vi "Query - DBL - 1D - Col.vi"(8 "error in":errorcluster, 10 "Query":string, 11 "Module ID":i32=-1) -> (0 "error out":errorcluster, 1 "Meta Data":variant, 2 "Return Data":dbl[](array[numeric]), 4 "Field Names":string[](array[string]))   [LabVIEW 2022 SP3, in "hse-db.lvlib" / "DB_CONNECTOR.lvlib"]
doc: "returns the first column\n\n____\nHAMPEL SOFTWARE ENGINEERING v1.4.0 (2023-12-19 09:52)"
uses:
  DB_CONNECTOR.lvlib
  hse-libraries/Source/hse-misc/Conversion/ConvertStringToFloat_Array-2D.vi
  hse-libraries/Source/hse-misc/hse-misc.lvlib
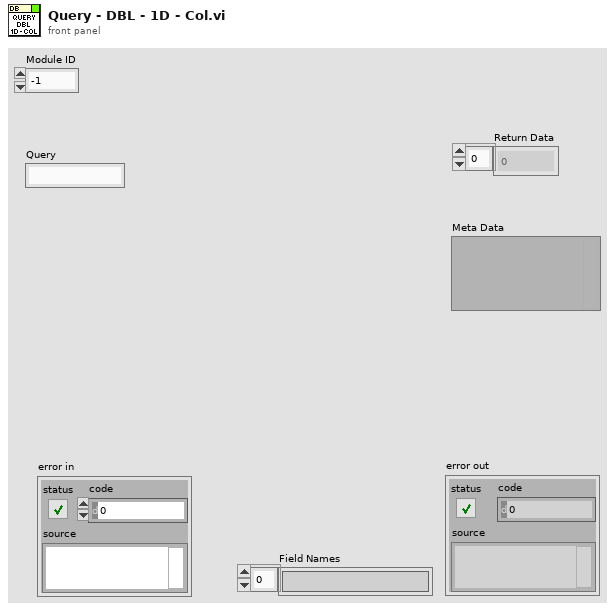
[diagram p1: front panel]
types:
  T1 = typedef "hse-db.lvlib/DB_CONNECTOR.lvlib/Query (Reply Payload)--cluster.ctl" = cluster{"Return Data":string[][], "Meta Data":variant, "Field Names":string[], "Query_error":errorcluster, "Module ID":i32}
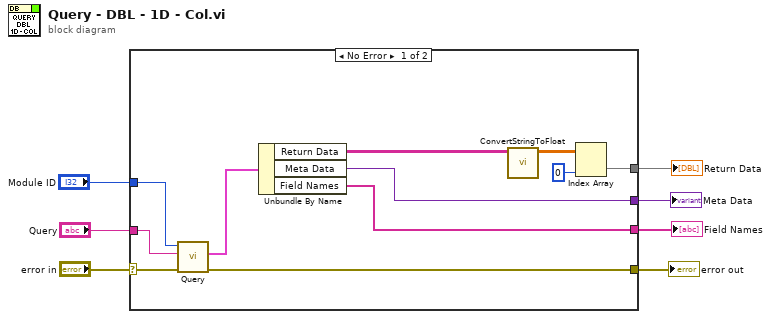
[diagram p0: block diagram]
diagram:
  n1 = case shown="No Error" "error in" {
    selector: "error in" -> [w13 w19]
    tunnel: [w12 w19] -> w6
    tunnel: "Query" -> [w10 _]
    tunnel: "Module ID" -> [w11 _]
    tunnel: [w17 _] -> w2
    tunnel: [w15 _] -> w3
    tunnel: [w14 _] -> w1
    frame No Error {
      n2 = call "Query.vi"("error in (no error)"=w13, "Query"=w10, "Module ID"=w11) -> ("error out"=w12:errorcluster, "Reply Payload"=w9:T1)  [unwired: 6 in, 1 out]
      n3 = Unbundle By Name(w9) -> ("Return Data"=w18:string[][], "Meta Data"=w17:variant, "Field Names"=w14:string[])
      n4 = call-poly "ConvertStringToFloat.vi"("String"=w18) -> ("Array of Doubles"=w16:dbl[][])  [unwired: 9 in, 1 out]
      n5 = Index Array(array=w16, index (col)=0 ("index (row)")) -> (element=w15:dbl[])  [unwired: 1 in]
    }
    frame Error {
    }
  }
  "error out" <- w6
  "Return Data" <- w3
  "Meta Data" <- w2
  "Field Names" <- w1
